vi "main3.vi"() -> ()   [LabVIEW 2011]
uses:
  genericVehicle.lvclass
  bus/bus.lvclass
  tricycle/tricycle.lvclass
panel:
  in  "Cluster":T1
  out "Array":dbl[](array[numeric])
  out "numberOfWheels 2":dbl
  in  "numberOfWheels":dbl
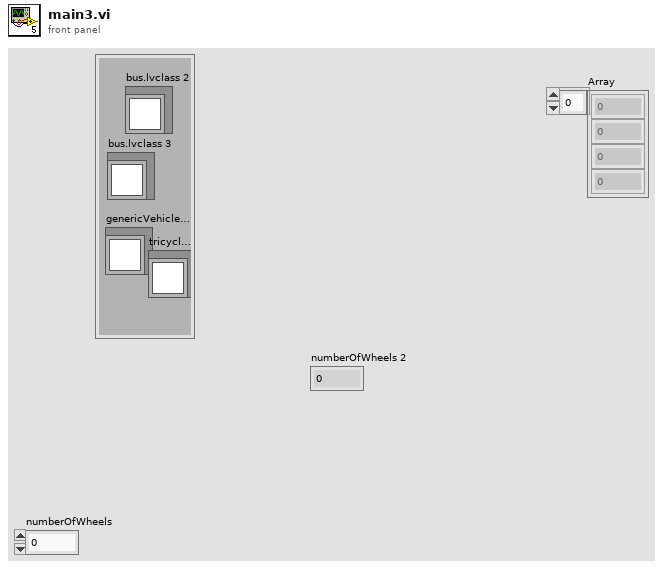
[diagram p1: front panel]
types:
  T1 = cluster{"genericVehicle.lvclass":refnum<class "genericVehicle.lvclass">, "bus.lvclass 2":refnum<class "bus.lvclass">, "bus.lvclass 3":refnum<class "bus.lvclass">, "tricycle.lvclass":refnum<class "tricycle.lvclass">}
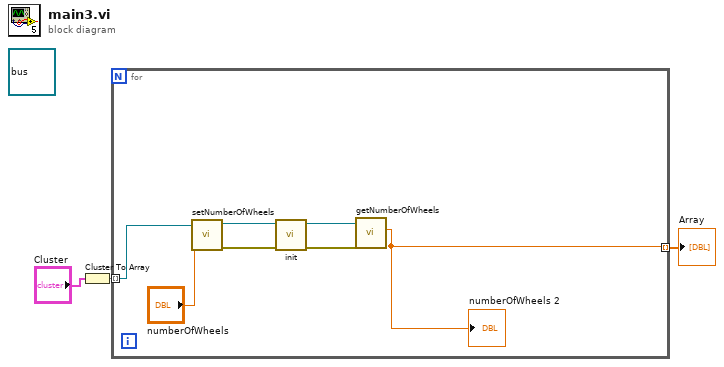
[diagram p0: block diagram]
diagram:
  (unwired) refnum<class "bus.lvclass"> refnum ("bus.lvclass")
  n1 = Cluster To Array(cluster="Cluster") -> (array=w3:refnum<class "genericVehicle.lvclass">[])
  n2 = for {
    tunnel: w3 -> [w5] mode=indexing
    tunnel: [w4] -> w2 mode=indexing
    n3 = call-dynamic "setNumberOfWheels.vi"("numberOfWheels"="numberOfWheels", "genericVehicle in"=w5) -> ("error out"=w7:errorcluster, "genericVehicle out"=w9:refnum<class "genericVehicle.lvclass">)  [unwired: 8 in]
    n4 = call-dynamic "init.vi"("error in (no error)"=w7, "genericVehicle in"=w9) -> ("error out"=w6:errorcluster, "genericVehicle out"=w8:refnum<class "genericVehicle.lvclass">)  [unwired: 8 in]
    n5 = call-dynamic "getNumberOfWheels.vi"("error in (no error)"=w6, "genericVehicle in"=w8) -> ("numberOfWheels"=w4:dbl)  [unwired: 7 in, 2 out]
    "numberOfWheels 2" <- w4
  }
  "Array" <- w2
